vi "Sunits.vi"(8 "error in (no error)":errorcluster, 11 "units":i32) -> (0 "error out":errorcluster, 3 "function return":string)   [LabVIEW 2023, in "POSCONV.lvlib"]
doc: "char *Sunits(int units);"
uses:
  POSCONV.lvlib
  C:/Users/J Gordon/Documents/Rail Tech/TV-HR/02 - Code/Modules/POSCONV/POSCONV.dll
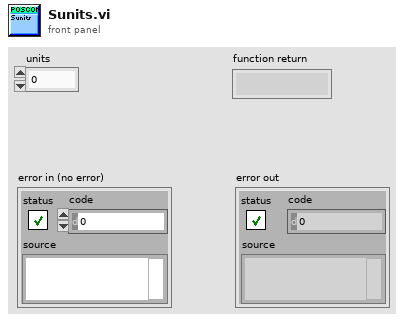
[diagram p1: front panel]
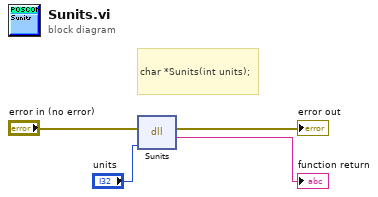
[diagram p0: block diagram]
diagram:
  # "char *Sunits(int units);"
  n1 = dll-call lib="C:/Users/J Gordon/Documents/Rail Tech/TV-HR/02 - Code/Modules/POSCONV/POSCONV.*" fn="Sunits"(error in="error in (no error)", "units"="units") -> (error out=→"error out":errorcluster, →"function return":string)  [unwired: 3 in, 1 out]
